vi "getTaskInfo.vi"   [LabVIEW 2015, in "pdbm_test_system.lvlib"]
uses:
  pdbm_test_system.lvlib
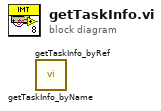
[diagram p0: block diagram]
diagram:
  n1 = call "getTaskInfo_byName.vi"() -> ()  [unwired: 8 in, 4 out]
  n2 = call "getTaskInfo_byRef.vi"() -> ()  [unwired: 8 in, 4 out]
